vi "PI_AreaScan_Prepare_1.vi"(0 "System":i32 min=0 max=3 step=1, 1 "Laser":string, 2 "Axis":string, 3 "da":dbl min=-100.0 max=100.0, 4 "db":dbl min=-100.0 max=100.0, 5 "error in (no error)":errorcluster caption="Fehler (Eingang, kein Fehler)", 6 "a0":dbl min=2.0 max=198.0 step=0.01, 8 "b0":dbl min=0.0 max=200.0 step=0.01, 9 "Resolution":dbl min=0.01 max=2.0 step=0.01, 10 "c0":dbl min=0.0 max=200.0 step=0.01, 11 "Pixel time":dbl) -> (14 "Tacq":dbl, 15 "lp":i32, 16 "ap":i32, 17 "Trigger":dbl[](array[numeric]), 19 "error out":errorcluster caption="Fehler (Ausgang)")   [LabVIEW 2009]
panel:
  out "ClockDivider":i32
  out "Amplitude":dbl format="%#_3g"
  out "Accelaration":dbl
  out "ttp":i32
  out "Scan lines":dbl
  out "slow axis":i32
  out "fast axis":i32
  out "Colors":i32
  out "Start position":dbl[](array[numeric])
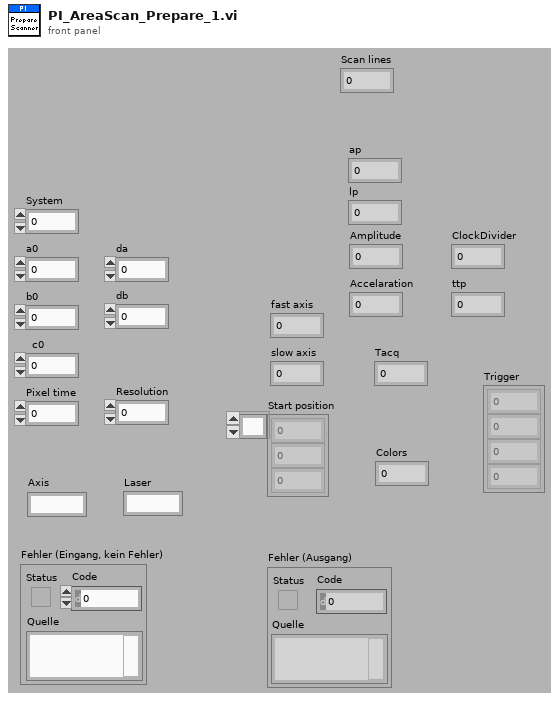
[diagram p1: front panel]
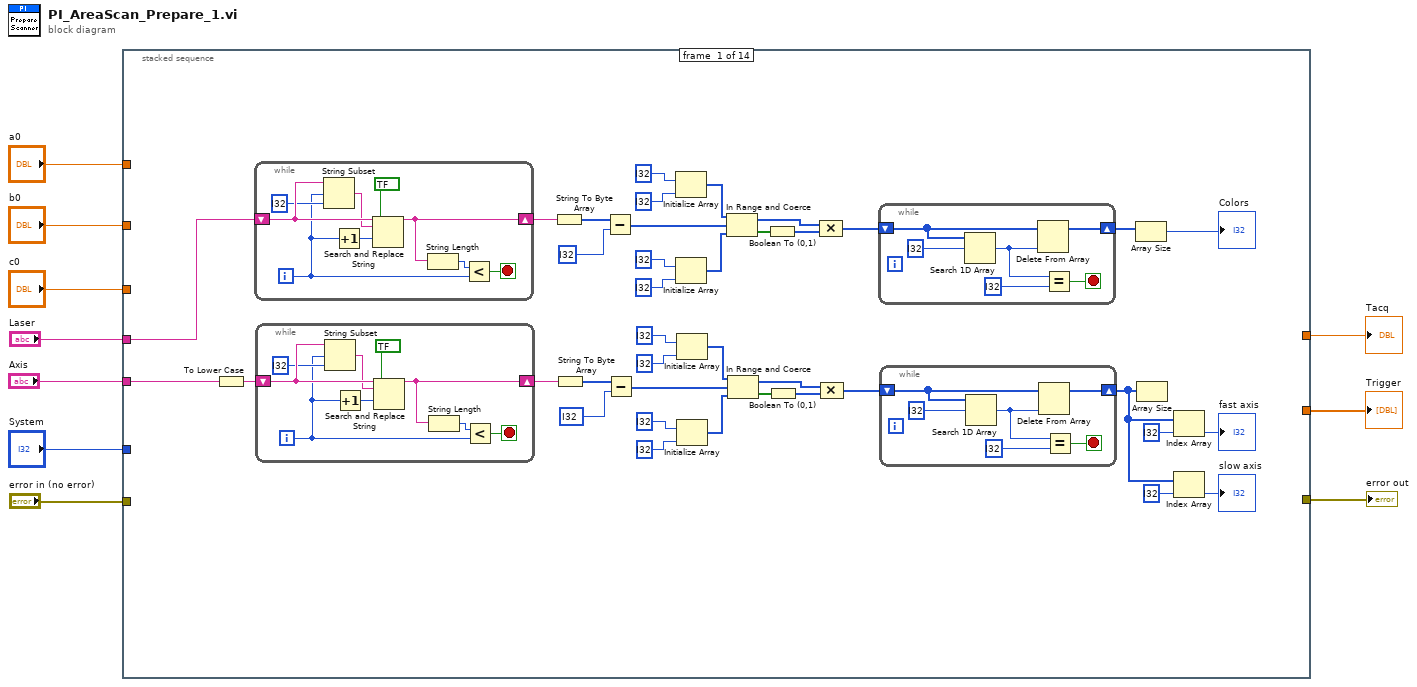
[diagram p0: block diagram]
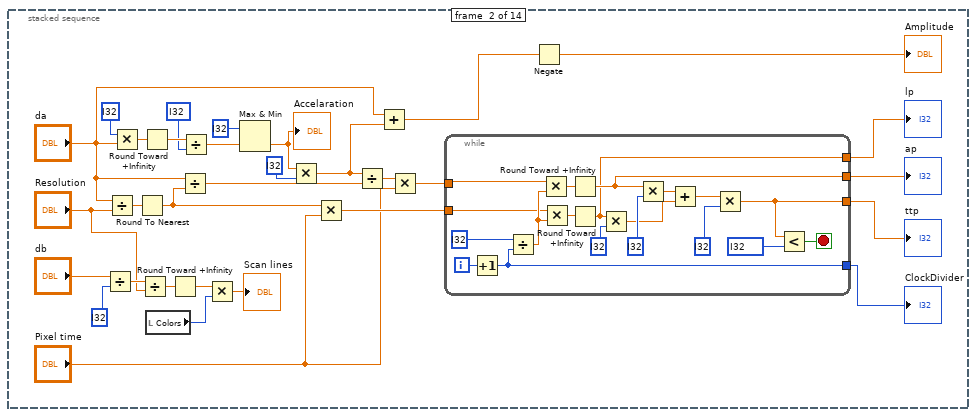
[diagram p2: hidden frame]
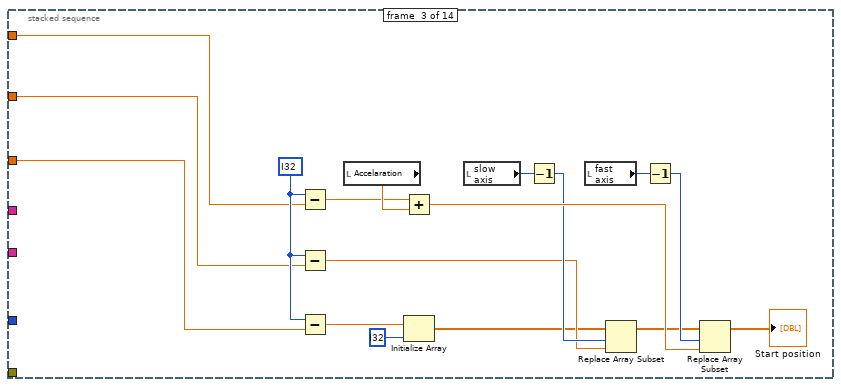
[diagram p3: hidden frame]
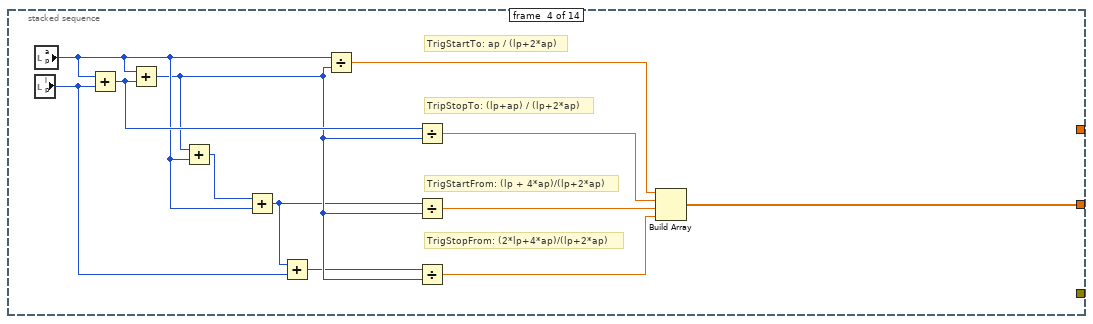
[diagram p4: hidden frame]
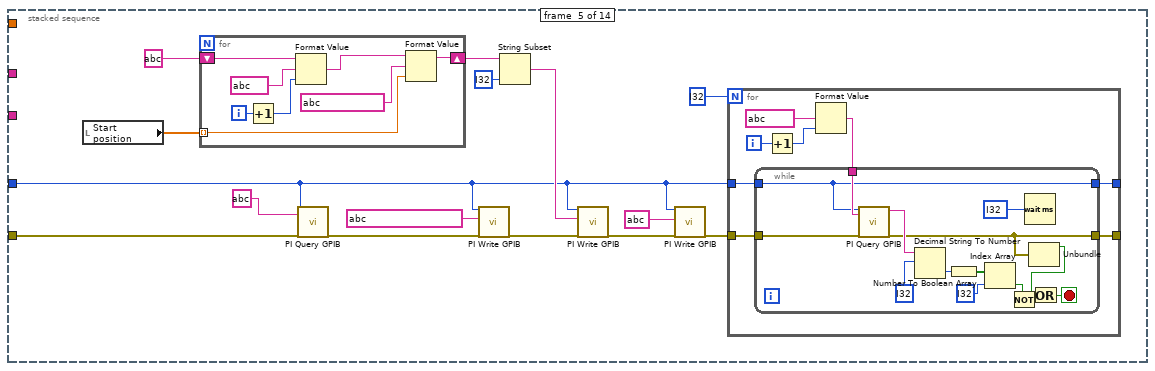
[diagram p5: hidden frame]
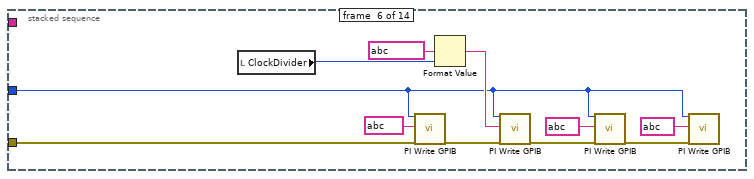
[diagram p6: hidden frame]
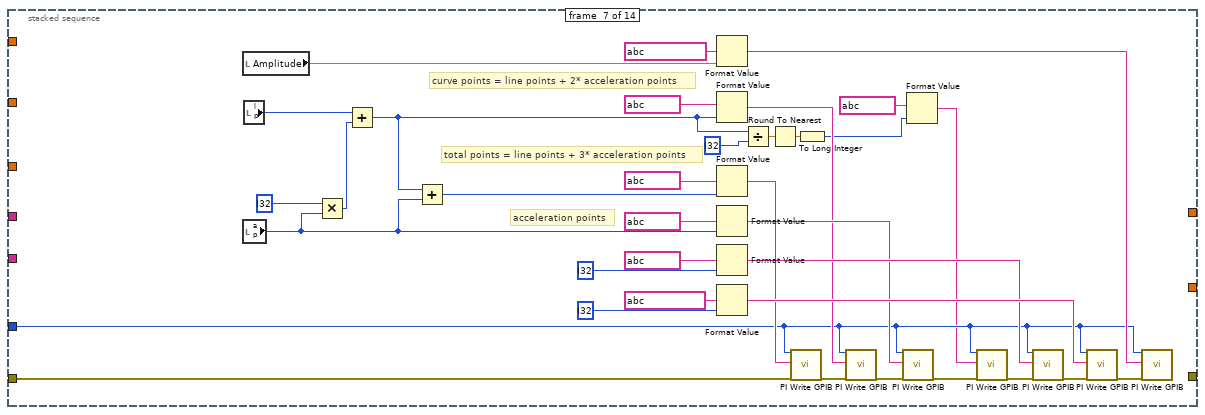
[diagram p7: hidden frame]
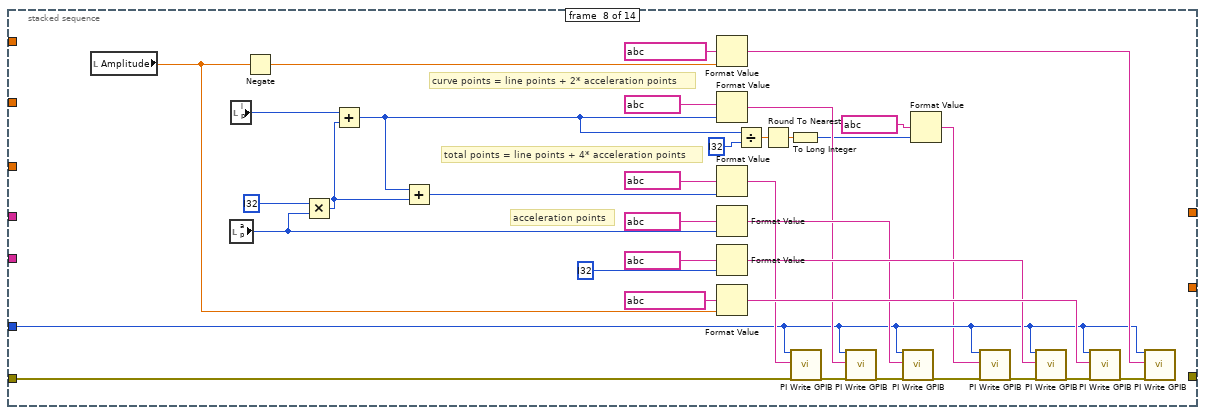
[diagram p8: hidden frame]
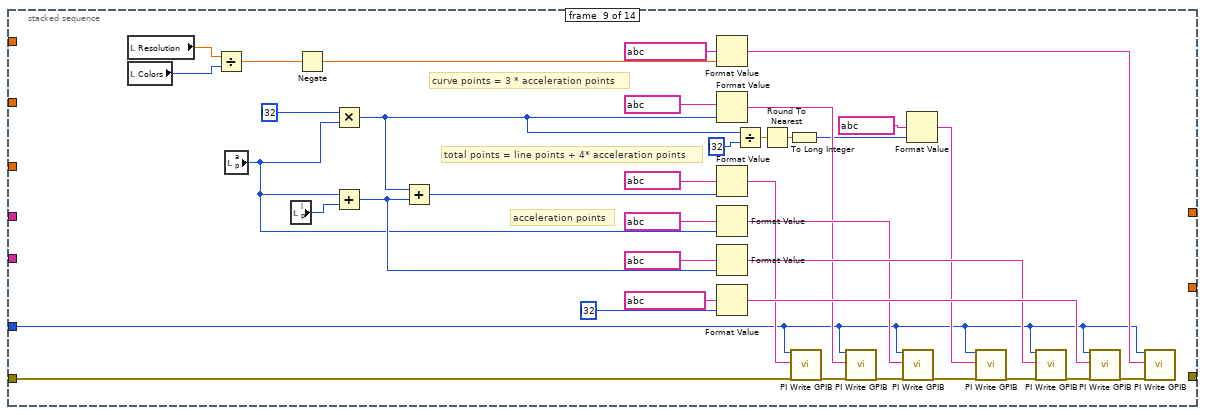
[diagram p9: hidden frame]
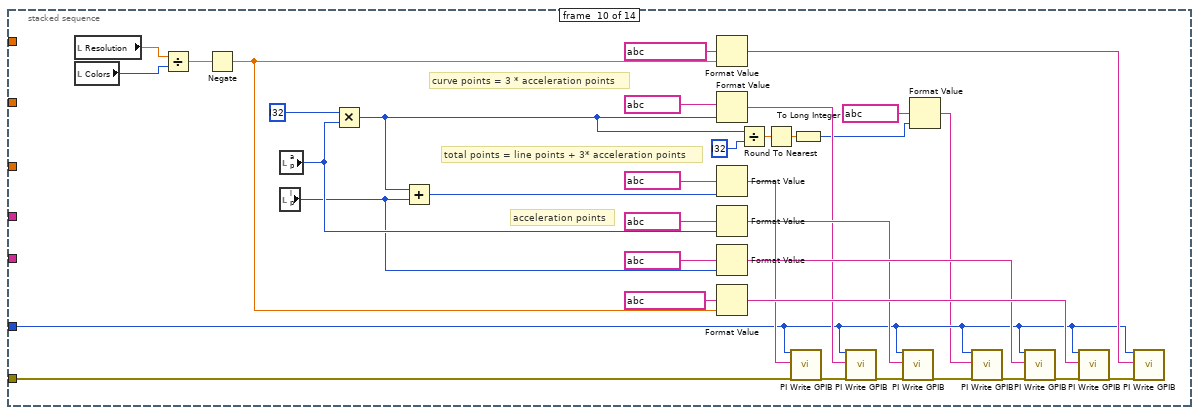
[diagram p10: hidden frame]
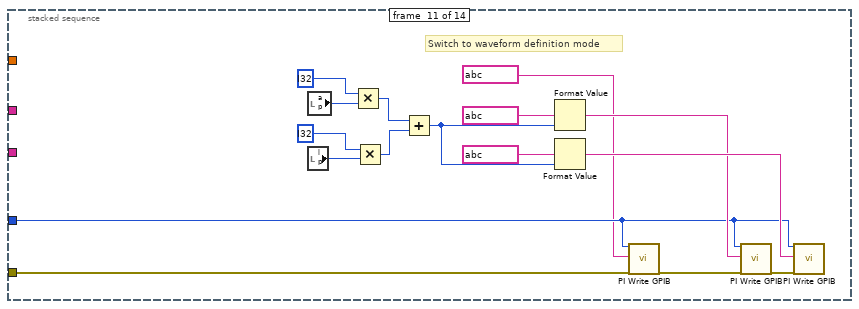
[diagram p11: hidden frame]
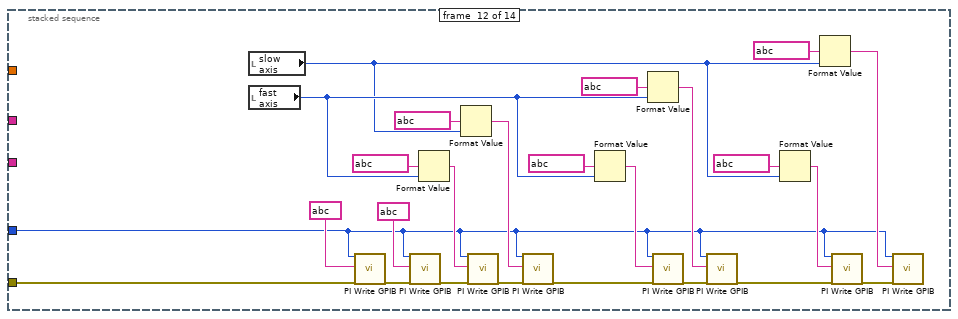
[diagram p12: hidden frame]
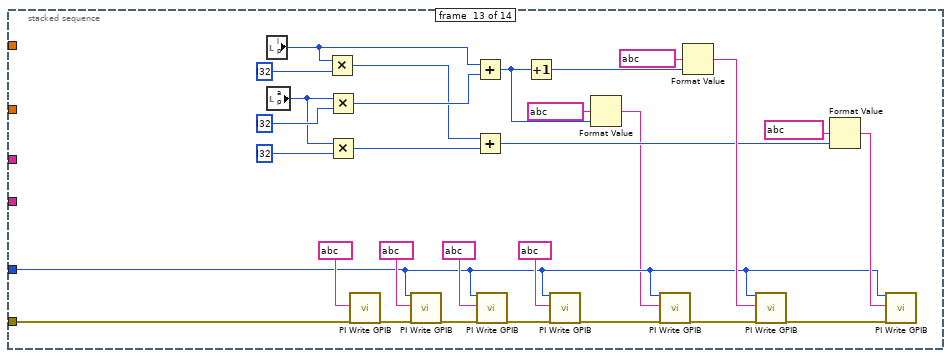
[diagram p13: hidden frame]
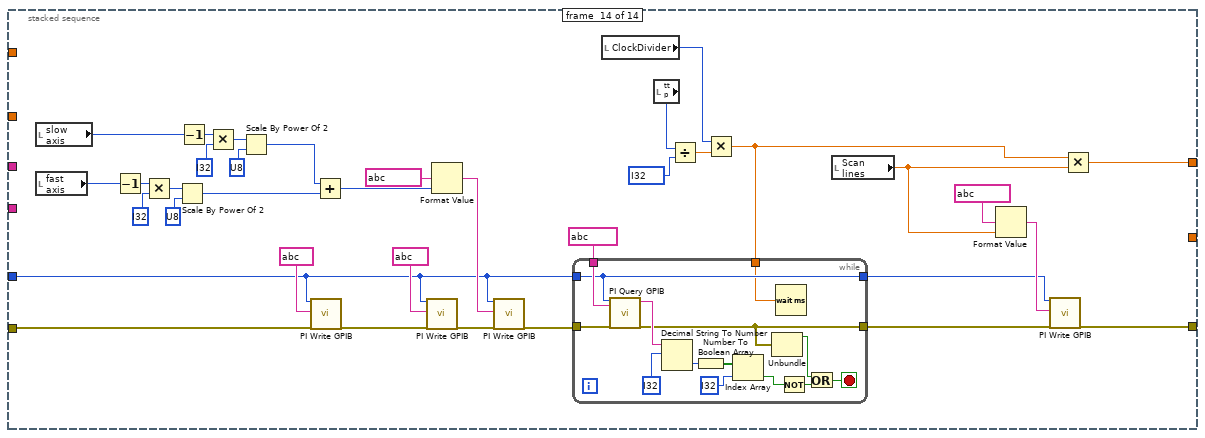
[diagram p14: hidden frame]
diagram:
  n1 = stacked-sequence {
    tunnel: "System" -> [_ _ _ _ w161 w203 w216 w254 w284 w324 w365 w372 w400 w427]
    tunnel: "error in (no error)" -> [_ _ _ _ w163 w204 w229 w266 w304 w339 w366 w373 w413 w428]
    tunnel: [_ _ _ _ _ _ _ _ _ _ _ _ _ w429] -> w8
    tunnel: "Laser" -> [w12 _ _ _ _ _ _ _ _ _ _ _ _ _]
    tunnel: "Axis" -> [w11 _ _ _ _ _ _ _ _ _ _ _ _ _]
    tunnel: "c0" -> [_ _ w131 _ _ _ _ _ _ _ _ _ _ _]
    tunnel: "b0" -> [_ _ w130 _ _ _ _ _ _ _ _ _ _ _]
    tunnel: "a0" -> [_ _ w129 _ _ _ _ _ _ _ _ _ _ _]
    tunnel: [_ _ _ _ _ _ _ _ _ _ _ _ _ w426] -> w2
    tunnel: [_ _ _ w146 _ _ _ _ _ _ _ _ _ _] -> w1
    frame #0 {
      n2 = To Lower Case(string=w11) -> (all lower case string=w19:string)
      n3 = while {
        shift-right: [w74] -> w39
        shift-left: w12 -> [w78]
        i -> [w70]
        stop <- w73 stop-if-true
        n4 = String Subset(string=w78, offset (0)=w70, length (rest)=i32 ?) -> (substring=w76:string)
        n5 = Increment(x=w70) -> (x+1=w71:i32)
        n6 = Search and Replace String(replace all?=bool ?, input string=w78, search string=w76, offset=w71) -> (result string=w74:string)  [unwired: 4 in, 3 out]
        n7 = String Length(string=w74) -> (length=w72:i32)
        n8 = Less?(x=w72, y=w70) -> (x < y?=w73:bool)
      }
      n9 = while {
        shift-right: [w59] -> w24
        shift-left: w19 -> [w63]
        i -> [w55]
        stop <- w58 stop-if-true
        n10 = String Subset(string=w63, offset (0)=w55, length (rest)=i32 ?) -> (substring=w61:string)
        n11 = Increment(x=w55) -> (x+1=w56:i32)
        n12 = Search and Replace String(replace all?=bool ?, input string=w63, search string=w61, offset=w56) -> (result string=w59:string)  [unwired: 4 in, 3 out]
        n13 = String Length(string=w59) -> (length=w57:i32)
        n14 = Less?(x=w57, y=w55) -> (x < y?=w58:bool)
      }
      n15 = String To Byte Array(string=w39) -> (unsigned byte array=w41:u8[])
      n16 = String To Byte Array(string=w24) -> (unsigned byte array=w26:u8[])
      n17 = Subtract(x=w41, y=i32 ?) -> (x-y=w38:i32[])
      n18 = Subtract(x=w26, y=i32 ?) -> (x-y=w23:i32[])
      n19 = Initialize Array(i32 ?, i32 ?) -> (w46:i32[])
      n20 = Initialize Array(i32 ?, i32 ?) -> (w43:i32[])
      n21 = Initialize Array(i32 ?, i32 ?) -> (w31:i32[])
      n22 = Initialize Array(i32 ?, i32 ?) -> (w28:i32[])
      n23 = In Range and Coerce(upper limit=w46, x=w38, lower limit=w43) -> (coerced(x)=w35:i32[], In Range?=w42:bool[])
      n24 = In Range and Coerce(upper limit=w31, x=w23, lower limit=w28) -> (coerced(x)=w20:i32[], In Range?=w27:bool[])
      n25 = Boolean To (0,1)(Boolean=w42) -> (0, 1=w36:i16[])
      n26 = Boolean To (0,1)(Boolean=w27) -> (0, 1=w21:i16[])
      n27 = Compound Arithmetic op=MULTIPLY(w35, w36) -> (w37:i32[])
      n28 = Compound Arithmetic op=MULTIPLY(w20, w21) -> (w22:i32[])
      n29 = while {
        shift-right: [w66] -> w34
        shift-left: w37 -> [w64]
        stop <- w67 stop-if-true
        n30 = Search 1D Array(1D array=w64, element=i32 ?) -> (index of element=w68:i32)  [unwired: 1 in]
        n31 = Delete From Array(array=w64, index=w68) -> (array with subset deleted=w66:i32[])  [unwired: 1 in, 1 out]
        n32 = Equal?(x=w68, y=i32 ?) -> (x = y?=w67:bool)
      }
      n33 = while {
        shift-right: [w51] -> w16
        shift-left: w22 -> [w49]
        stop <- w52 stop-if-true
        n34 = Search 1D Array(1D array=w49, element=i32 ?) -> (index of element=w53:i32)  [unwired: 1 in]
        n35 = Delete From Array(array=w49, index=w53) -> (array with subset deleted=w51:i32[])  [unwired: 1 in, 1 out]
        n36 = Equal?(x=w53, y=i32 ?) -> (x = y?=w52:bool)
      }
      n37 = Array Size(array=w34) -> (size(s)=→"Colors":i32)
      n38 = Array Size(array=w16) -> ()  [unwired: 1 out]
      n39 = Index Array(array=w16, index=i32 ?) -> (element=→"fast axis":i32)
      n40 = Index Array(array=w16, index=i32 ?) -> (element=→"slow axis":i32)
    }
    frame #1 {
      n41 = Divide(x="db", y=i32 ?) -> (x/y=w101:dbl)
      n42 = Divide(x="da", y="Resolution") -> (x/y=w103:dbl)
      n43 = Multiply(x=i32 ?, y="da") -> (x*y=w108:dbl)
      n44 = Round To Nearest(number=w103) -> (nearest integer value=w90:dbl)
      n45 = Divide(x=w101, y="Resolution") -> (x/y=w95:dbl)
      n46 = Round Toward +Infinity(x=w108) -> (ceil(x): smallest int >= x=w107:dbl)
      n47 = local read "Colors"() -> (w98:i32)
      n48 = Round Toward +Infinity(x=w95) -> (ceil(x): smallest int >= x=w96:dbl)
      n49 = Divide(x="da", y=w90) -> (x/y=w89:dbl)
      n50 = Divide(x=w107, y=i32 ?) -> (x/y=w105:dbl)
      n51 = Multiply(x=w96, y=w98) -> (x*y=→"Scan lines":dbl)
      n52 = Max & Min(x=i32 ?, y=w105) -> (min(x,y)=w86:dbl)  [unwired: 1 out]
      "Accelaration" <- w86
      n53 = Multiply(x=w86, y=i32 ?) -> (x*y=w88:dbl)
      n54 = Multiply(x=w90, y="Pixel time") -> (x*y=w94:dbl)
      n55 = Divide(x=w88, y=w89) -> (x/y=w91:dbl)
      n56 = Add(x="da", y=w88) -> (x+y=w80:dbl)
      n57 = Multiply(x=w91, y="Pixel time") -> (x*y=w92:dbl)
      n58 = while {
        tunnel: w94 -> [w125]
        tunnel: w92 -> [w124]
        tunnel: [w113] -> w84
        tunnel: [w112] -> w81
        tunnel: [w111] -> w83
        tunnel: [w110] -> w82
        i -> [w128]
        stop <- w114 stop-if-true
        n59 = Increment(x=w128) -> (x+1=w112:i32)
        n60 = Divide(x=i32 ?, y=w112) -> (x/y=w126:dbl)
        n61 = Multiply(x=w124, y=w126) -> (x*y=w123:dbl)
        n62 = Multiply(x=w125, y=w126) -> (x*y=w122:dbl)
        n63 = Round Toward +Infinity(x=w123) -> (ceil(x): smallest int >= x=w111:dbl)
        n64 = Round Toward +Infinity(x=w122) -> (ceil(x): smallest int >= x=w110:dbl)
        n65 = Multiply(x=w110, y=i32 ?) -> (x*y=w118:dbl)
        n66 = Multiply(x=w111, y=i32 ?) -> (x*y=w119:dbl)
        n67 = Add(x=w119, y=w118) -> (x+y=w117:dbl)
        n68 = Multiply(x=w117, y=i32 ?) -> (x*y=w113:dbl)
        n69 = Less?(x=w113, y=i32 ?) -> (x < y?=w114:bool)
      }
      "ttp" <- w84
      "ap" <- w83
      "lp" <- w82
      "ClockDivider" <- w81
      n70 = Negate(x=w80) -> (-x=→"Amplitude":dbl)
    }
    frame #2 {
      w132 = i32 ?
      n71 = Subtract(x=w132, y=w129) -> (x-y=w140:dbl)
      n72 = Subtract(x=w132, y=w130) -> (x-y=w136:dbl)
      n73 = Subtract(x=w132, y=w131) -> (x-y=w134:dbl)
      n74 = local read "Accelaration"() -> (w142:dbl)
      n75 = Add(x=w140, y=w142) -> (x+y=w141:dbl)
      n76 = Initialize Array(w134, i32 ?) -> (w135:dbl[])
      n77 = local read "slow axis"() -> (w145:i32)
      n78 = Decrement(x=w145) -> (x-1=w138:i32)
      n79 = local read "fast axis"() -> (w144:i32)
      n80 = Replace Array Subset(array=w135, new element=w136, index=w138) -> (w137:dbl[])
      n81 = Decrement(x=w144) -> (x-1=w139:i32)
      n82 = Replace Array Subset(array=w137, new element=w141, index=w139) -> (→"Start position":dbl[])
    }
    frame #3 {
      # "TrigStopFrom: (2*lp+4*ap)/(lp+2*ap)"
      # "TrigStartFrom: (lp + 4*ap)/(lp+2*ap)"
      # "TripStopTo: (lp+ap) / (lp+2*ap)"
      # "TrigStartTo: ap / (lp+2*ap)"
      n83 = local read "ap"() -> (w152:i32)
      n84 = local read "lp"() -> (w148:i32)
      n85 = Add(x=w152, y=w148) -> (x+y=w153:i32)
      n86 = Add(x=w152, y=w153) -> (x+y=w151:i32)
      n87 = Add(x=w151, y=w152) -> (x+y=w150:i32)
      n88 = Add(x=w150, y=w152) -> (x+y=w147:i32)
      n89 = Add(x=w147, y=w148) -> (x+y=w149:i32)
      n90 = Divide(x=w152, y=w151) -> (x/y=w154:dbl)
      n91 = Divide(x=w153, y=w151) -> (x/y=w155:dbl)
      n92 = Divide(x=w147, y=w151) -> (x/y=w156:dbl)
      n93 = Divide(x=w149, y=w151) -> (x/y=w157:dbl)
      n94 = Build Array(w154, w155, w156, w157) -> (w146:dbl[])
    }
    frame #4 {
      n95 = local read "Start position"() -> (w160:dbl[])
      n96 = for {
        shift-right: [w200] -> w170
        shift-left: string ? -> [w202]
        tunnel: w160 -> [w195] mode=indexing
        i -> [w197]
        n97 = Increment(x=w197) -> (x+1=w196:i32)
        n98 = Format Value(string ("")=w202, format string=string ?, value (0)=w196) -> (output string=w201:string)
        n99 = Format Value(string ("")=w201, format string=string ?, value (0)=w195) -> (output string=w200:string)
      }
      n100 = call "PI Query GPIB.vi"("System no."=w161, "String to send"=string ?, "error in"=w163) -> ("error out"=w168:errorcluster)  [unwired: 14 in, 2 out]
      n101 = call "PI Write GPIB.vi"("System no."=w161, "String to send"=string ?, "error in"=w168) -> ("error out"=w164:errorcluster)  [unwired: 16 in]
      n102 = String Subset(string=w170, length (rest)=i32 ?) -> (substring=w172:string)  [unwired: 1 in]
      n103 = call "PI Write GPIB.vi"("System no."=w161, "String to send"=w172, "error in"=w164) -> ("error out"=w166:errorcluster)  [unwired: 16 in]
      n104 = call "PI Write GPIB.vi"("System no."=w161, "String to send"=string ?, "error in"=w166) -> ("error out"=w165:errorcluster)  [unwired: 16 in]
      n105 = for {
        N: i32 ? -> [_]
        tunnel: w165 -> [w176]
        tunnel: w161 -> [w175]
        tunnel: [w174] -> _
        tunnel: [w173] -> _
        i -> [w180]
        n106 = Increment(x=w180) -> (x+1=w179:i32)
        n107 = Format Value(format string=string ?, value (0)=w179) -> (output string=w177:string)  [unwired: 1 in]
        n108 = while {
          tunnel: w177 -> [w194]
          tunnel: w176 -> [w193]
          tunnel: w175 -> [w189]
          tunnel: [w188] -> w174
          tunnel: [w189] -> w173
          stop <- w183 stop-if-true
          n109 = call "PI Query GPIB.vi"("System no."=w189, "String to send"=w194, "error in"=w193) -> ("String read"=w191:string, "error out"=w188:errorcluster)  [unwired: 14 in, 1 out]
          n110 = Decimal String To Number(string=w191, offset=i32 ?) -> (number=w190:i32)  [unwired: 1 in, 1 out]
          n111 = Number To Boolean Array(number=w190) -> (Boolean array=w185:bool[])
          n112 = Index Array(array=w185, index=i32 ?) -> (element=w184:bool)
          n113 = Not(x=w184) -> (.not. x?=w181:bool)
          n114 = Wait (ms)(milliseconds to wait=i32 ?) -> ()  [unwired: 1 out]
          n115 = Unbundle(w188) -> ("status"=w187:bool)  [unwired: 2 out]
          n116 = Or(x=w187, y=w181) -> (x .or. y?=w183:bool)
        }
      }
    }
    frame #5 {
      n117 = local read "ClockDivider"() -> (w213:i32)
      n118 = call "PI Write GPIB.vi"("System no."=w203, "String to send"=string ?, "error in"=w204) -> ("error out"=w205:errorcluster)  [unwired: 16 in]
      n119 = Format Value(format string=string ?, value (0)=w213) -> (output string=w210:string)  [unwired: 1 in]
      n120 = call "PI Write GPIB.vi"("System no."=w203, "String to send"=w210, "error in"=w205) -> ("error out"=w207:errorcluster)  [unwired: 16 in]
      n121 = call "PI Write GPIB.vi"("System no."=w203, "String to send"=string ?, "error in"=w207) -> ("error out"=w208:errorcluster)  [unwired: 16 in]
      n122 = call "PI Write GPIB.vi"("System no."=w203, "String to send"=string ?, "error in"=w208) -> ()  [unwired: 16 in, 1 out]
    }
    frame #6 {
      # "acceleration points"
      # "total points = line points + 3* acceleration points"
      # "curve points = line points + 2* acceleration points"
      n123 = local read "Amplitude"() -> (w214:dbl)
      n124 = local read "ap"() -> (w225:i32)
      n125 = local read "lp"() -> (w227:i32)
      n126 = Multiply(x=i32 ?, y=w225) -> (x*y=w228:i32)
      n127 = Add(x=w227, y=w228) -> (x+y=w222:i32)
      n128 = Add(x=w222, y=w225) -> (x+y=w226:i32)
      n129 = Format Value(format string=string ?, value (0)=w214) -> (output string=w247:string)  [unwired: 1 in]
      n130 = Format Value(format string=string ?, value (0)=w222) -> (output string=w243:string)  [unwired: 1 in]
      n131 = Format Value(format string=string ?, value (0)=w226) -> (output string=w242:string)  [unwired: 1 in]
      n132 = Format Value(format string=string ?, value (0)=w225) -> (output string=w244:string)  [unwired: 1 in]
      n133 = Format Value(format string=string ?, value (0)=i32 ?) -> (output string=w245:string)  [unwired: 1 in]
      n134 = Format Value(format string=string ?, value (0)=i32 ?) -> (output string=w246:string)  [unwired: 1 in]
      n135 = Divide(x=w222, y=i32 ?) -> (x/y=w221:dbl)
      n136 = Round To Nearest(number=w221) -> (nearest integer value=w218:dbl)
      n137 = call "PI Write GPIB.vi"("System no."=w216, "String to send"=w242, "error in"=w229) -> ("error out"=w241:errorcluster)  [unwired: 16 in]
      n138 = To Long Integer(number=w218) -> (32bit integer=w219:i32)
      n139 = call "PI Write GPIB.vi"("System no."=w216, "String to send"=w243, "error in"=w241) -> ("error out"=w248:errorcluster)  [unwired: 16 in]
      n140 = call "PI Write GPIB.vi"("System no."=w216, "String to send"=w244, "error in"=w248) -> ("error out"=w238:errorcluster)  [unwired: 16 in]
      n141 = Format Value(format string=string ?, value (0)=w219) -> (output string=w215:string)  [unwired: 1 in]
      n142 = call "PI Write GPIB.vi"("System no."=w216, "String to send"=w215, "error in"=w238) -> ("error out"=w217:errorcluster)  [unwired: 16 in]
      n143 = call "PI Write GPIB.vi"("System no."=w216, "String to send"=w245, "error in"=w217) -> ("error out"=w239:errorcluster)  [unwired: 16 in]
      n144 = call "PI Write GPIB.vi"("System no."=w216, "String to send"=w246, "error in"=w239) -> ("error out"=w240:errorcluster)  [unwired: 16 in]
      n145 = call "PI Write GPIB.vi"("System no."=w216, "String to send"=w247, "error in"=w240) -> ()  [unwired: 16 in, 1 out]
    }
    frame #7 {
      # "acceleration points"
      # "total points = line points + 4* acceleration points"
      # "curve points = line points + 2* acceleration points"
      n146 = local read "Amplitude"() -> (w250:dbl)
      n147 = local read "ap"() -> (w263:i32)
      n148 = local read "lp"() -> (w265:i32)
      n149 = Negate(x=w250) -> (-x=w249:dbl)
      n150 = Multiply(x=i32 ?, y=w263) -> (x*y=w262:i32)
      n151 = Add(x=w265, y=w262) -> (x+y=w252:i32)
      n152 = Add(x=w252, y=w262) -> (x+y=w264:i32)
      n153 = Format Value(format string=string ?, value (0)=w249) -> (output string=w282:string)  [unwired: 1 in]
      n154 = Format Value(format string=string ?, value (0)=w252) -> (output string=w278:string)  [unwired: 1 in]
      n155 = Format Value(format string=string ?, value (0)=w264) -> (output string=w277:string)  [unwired: 1 in]
      n156 = Format Value(format string=string ?, value (0)=w263) -> (output string=w279:string)  [unwired: 1 in]
      n157 = Format Value(format string=string ?, value (0)=i32 ?) -> (output string=w280:string)  [unwired: 1 in]
      n158 = Format Value(format string=string ?, value (0)=w250) -> (output string=w281:string)  [unwired: 1 in]
      n159 = Divide(x=w252, y=i32 ?) -> (x/y=w260:dbl)
      n160 = Round To Nearest(number=w260) -> (nearest integer value=w257:dbl)
      n161 = To Long Integer(number=w257) -> (32bit integer=w258:i32)
      n162 = call "PI Write GPIB.vi"("System no."=w254, "String to send"=w277, "error in"=w266) -> ("error out"=w276:errorcluster)  [unwired: 16 in]
      n163 = call "PI Write GPIB.vi"("System no."=w254, "String to send"=w278, "error in"=w276) -> ("error out"=w283:errorcluster)  [unwired: 16 in]
      n164 = call "PI Write GPIB.vi"("System no."=w254, "String to send"=w279, "error in"=w283) -> ("error out"=w256:errorcluster)  [unwired: 16 in]
      n165 = Format Value(format string=string ?, value (0)=w258) -> (output string=w253:string)  [unwired: 1 in]
      n166 = call "PI Write GPIB.vi"("System no."=w254, "String to send"=w253, "error in"=w256) -> ("error out"=w255:errorcluster)  [unwired: 16 in]
      n167 = call "PI Write GPIB.vi"("System no."=w254, "String to send"=w280, "error in"=w255) -> ("error out"=w274:errorcluster)  [unwired: 16 in]
      n168 = call "PI Write GPIB.vi"("System no."=w254, "String to send"=w281, "error in"=w274) -> ("error out"=w275:errorcluster)  [unwired: 16 in]
      n169 = call "PI Write GPIB.vi"("System no."=w254, "String to send"=w282, "error in"=w275) -> ()  [unwired: 16 in, 1 out]
    }
    frame #8 {
      # "acceleration points"
      # "total points = line points + 4* acceleration points"
      # "curve points = 3 * acceleration points"
      n170 = local read "Resolution"() -> (w302:dbl)
      n171 = local read "Colors"() -> (w299:i32)
      n172 = Divide(x=w302, y=w299) -> (x/y=w300:dbl)
      n173 = local read "ap"() -> (w294:i32)
      n174 = local read "lp"() -> (w297:i32)
      n175 = Negate(x=w300) -> (-x=w298:dbl)
      n176 = Multiply(x=i32 ?, y=w294) -> (x*y=w289:i32)
      n177 = Add(x=w294, y=w297) -> (x+y=w295:i32)
      n178 = Add(x=w289, y=w295) -> (x+y=w303:i32)
      n179 = Format Value(format string=string ?, value (0)=w298) -> (output string=w319:string)  [unwired: 1 in]
      n180 = Format Value(format string=string ?, value (0)=w289) -> (output string=w315:string)  [unwired: 1 in]
      n181 = Format Value(format string=string ?, value (0)=w303) -> (output string=w314:string)  [unwired: 1 in]
      n182 = Format Value(format string=string ?, value (0)=w294) -> (output string=w316:string)  [unwired: 1 in]
      n183 = Format Value(format string=string ?, value (0)=w295) -> (output string=w317:string)  [unwired: 1 in]
      n184 = Format Value(format string=string ?, value (0)=i32 ?) -> (output string=w318:string)  [unwired: 1 in]
      n185 = Divide(x=w289, y=i32 ?) -> (x/y=w293:dbl)
      n186 = Round To Nearest(number=w293) -> (nearest integer value=w290:dbl)
      n187 = To Long Integer(number=w290) -> (32bit integer=w291:i32)
      n188 = call "PI Write GPIB.vi"("System no."=w284, "String to send"=w314, "error in"=w304) -> ("error out"=w313:errorcluster)  [unwired: 16 in]
      n189 = call "PI Write GPIB.vi"("System no."=w284, "String to send"=w315, "error in"=w313) -> ("error out"=w320:errorcluster)  [unwired: 16 in]
      n190 = call "PI Write GPIB.vi"("System no."=w284, "String to send"=w316, "error in"=w320) -> ("error out"=w286:errorcluster)  [unwired: 16 in]
      n191 = Format Value(format string=string ?, value (0)=w291) -> (output string=w287:string)  [unwired: 1 in]
      n192 = call "PI Write GPIB.vi"("System no."=w284, "String to send"=w287, "error in"=w286) -> ("error out"=w285:errorcluster)  [unwired: 16 in]
      n193 = call "PI Write GPIB.vi"("System no."=w284, "String to send"=w317, "error in"=w285) -> ("error out"=w311:errorcluster)  [unwired: 16 in]
      n194 = call "PI Write GPIB.vi"("System no."=w284, "String to send"=w318, "error in"=w311) -> ("error out"=w312:errorcluster)  [unwired: 16 in]
      n195 = call "PI Write GPIB.vi"("System no."=w284, "String to send"=w319, "error in"=w312) -> ()  [unwired: 16 in, 1 out]
    }
    frame #9 {
      # "acceleration points"
      # "total points = line points + 3* acceleration points"
      # "curve points = 3 * acceleration points"
      n196 = local read "Resolution"() -> (w337:dbl)
      n197 = local read "Colors"() -> (w336:i32)
      n198 = Divide(x=w337, y=w336) -> (x/y=w333:dbl)
      n199 = Negate(x=w333) -> (-x=w331:dbl)
      n200 = local read "ap"() -> (w334:i32)
      n201 = local read "lp"() -> (w332:i32)
      n202 = Multiply(x=i32 ?, y=w334) -> (x*y=w322:i32)
      n203 = Add(x=w322, y=w332) -> (x+y=w338:i32)
      n204 = Format Value(format string=string ?, value (0)=w331) -> (output string=w354:string)  [unwired: 1 in]
      n205 = Format Value(format string=string ?, value (0)=w322) -> (output string=w350:string)  [unwired: 1 in]
      n206 = Format Value(format string=string ?, value (0)=w338) -> (output string=w349:string)  [unwired: 1 in]
      n207 = Format Value(format string=string ?, value (0)=w334) -> (output string=w351:string)  [unwired: 1 in]
      n208 = Format Value(format string=string ?, value (0)=w332) -> (output string=w352:string)  [unwired: 1 in]
      n209 = Format Value(format string=string ?, value (0)=w331) -> (output string=w353:string)  [unwired: 1 in]
      n210 = Divide(x=w322, y=i32 ?) -> (x/y=w330:dbl)
      n211 = Round To Nearest(number=w330) -> (nearest integer value=w327:dbl)
      n212 = call "PI Write GPIB.vi"("System no."=w324, "String to send"=w349, "error in"=w339) -> ("error out"=w348:errorcluster)  [unwired: 16 in]
      n213 = To Long Integer(number=w327) -> (32bit integer=w328:i32)
      n214 = call "PI Write GPIB.vi"("System no."=w324, "String to send"=w350, "error in"=w348) -> ("error out"=w355:errorcluster)  [unwired: 16 in]
      n215 = call "PI Write GPIB.vi"("System no."=w324, "String to send"=w351, "error in"=w355) -> ("error out"=w326:errorcluster)  [unwired: 16 in]
      n216 = Format Value(format string=string ?, value (0)=w328) -> (output string=w323:string)  [unwired: 1 in]
      n217 = call "PI Write GPIB.vi"("System no."=w324, "String to send"=w323, "error in"=w326) -> ("error out"=w325:errorcluster)  [unwired: 16 in]
      n218 = call "PI Write GPIB.vi"("System no."=w324, "String to send"=w352, "error in"=w325) -> ("error out"=w346:errorcluster)  [unwired: 16 in]
      n219 = call "PI Write GPIB.vi"("System no."=w324, "String to send"=w353, "error in"=w346) -> ("error out"=w347:errorcluster)  [unwired: 16 in]
      n220 = call "PI Write GPIB.vi"("System no."=w324, "String to send"=w354, "error in"=w347) -> ()  [unwired: 16 in, 1 out]
    }
    frame #10 {
      # "Switch to waveform definition mode"
      n221 = local read "ap"() -> (w361:i32)
      n222 = local read "lp"() -> (w362:i32)
      n223 = Multiply(x=i32 ?, y=w361) -> (x*y=w358:i32)
      n224 = Multiply(x=i32 ?, y=w362) -> (x*y=w357:i32)
      n225 = Add(x=w358, y=w357) -> (x+y=w356:i32)
      n226 = Format Value(format string=string ?, value (0)=w356) -> (output string=w370:string)  [unwired: 1 in]
      n227 = Format Value(format string=string ?, value (0)=w356) -> (output string=w371:string)  [unwired: 1 in]
      n228 = call "PI Write GPIB.vi"("System no."=w365, "String to send"=string ?, "error in"=w366) -> ("error out"=w363:errorcluster)  [unwired: 16 in]
      n229 = call "PI Write GPIB.vi"("System no."=w365, "String to send"=w370, "error in"=w363) -> ("error out"=w369:errorcluster)  [unwired: 16 in]
      n230 = call "PI Write GPIB.vi"("System no."=w365, "String to send"=w371, "error in"=w369) -> ()  [unwired: 16 in, 1 out]
    }
    frame #11 {
      n231 = local read "slow axis"() -> (w387:i32)
      n232 = local read "fast axis"() -> (w388:i32)
      n233 = call "PI Write GPIB.vi"("System no."=w372, "String to send"=string ?, "error in"=w373) -> ("error out"=w379:errorcluster)  [unwired: 16 in]
      n234 = call "PI Write GPIB.vi"("System no."=w372, "String to send"=string ?, "error in"=w379) -> ("error out"=w374:errorcluster)  [unwired: 16 in]
      n235 = Format Value(format string=string ?, value (0)=w388) -> (output string=w391:string)  [unwired: 1 in]
      n236 = Format Value(format string=string ?, value (0)=w387) -> (output string=w392:string)  [unwired: 1 in]
      n237 = call "PI Write GPIB.vi"("System no."=w372, "String to send"=w391, "error in"=w374) -> ("error out"=w375:errorcluster)  [unwired: 16 in]
      n238 = call "PI Write GPIB.vi"("System no."=w372, "String to send"=w392, "error in"=w375) -> ("error out"=w376:errorcluster)  [unwired: 16 in]
      n239 = Format Value(format string=string ?, value (0)=w388) -> (output string=w393:string)  [unwired: 1 in]
      n240 = Format Value(format string=string ?, value (0)=w388) -> (output string=w394:string)  [unwired: 1 in]
      n241 = call "PI Write GPIB.vi"("System no."=w372, "String to send"=w393, "error in"=w376) -> ("error out"=w377:errorcluster)  [unwired: 16 in]
      n242 = call "PI Write GPIB.vi"("System no."=w372, "String to send"=w394, "error in"=w377) -> ("error out"=w378:errorcluster)  [unwired: 16 in]
      n243 = Format Value(format string=string ?, value (0)=w387) -> (output string=w395:string)  [unwired: 1 in]
      n244 = Format Value(format string=string ?, value (0)=w387) -> (output string=w396:string)  [unwired: 1 in]
      n245 = call "PI Write GPIB.vi"("System no."=w372, "String to send"=w395, "error in"=w378) -> ("error out"=w386:errorcluster)  [unwired: 16 in]
      n246 = call "PI Write GPIB.vi"("System no."=w372, "String to send"=w396, "error in"=w386) -> ()  [unwired: 16 in, 1 out]
    }
    frame #12 {
      n247 = local read "lp"() -> (w407:i32)
      n248 = local read "ap"() -> (w409:i32)
      n249 = Multiply(x=w407, y=i32 ?) -> (x*y=w405:i32)
      n250 = Multiply(x=w409, y=i32 ?) -> (x*y=w412:i32)
      n251 = Multiply(x=w409, y=i32 ?) -> (x*y=w406:i32)
      n252 = call "PI Write GPIB.vi"("String to send"=string ?, "error in"=w413) -> ("error out"=w415:errorcluster)  [unwired: 17 in]
      n253 = call "PI Write GPIB.vi"("System no."=w400, "String to send"=string ?, "error in"=w415) -> ("error out"=w414:errorcluster)  [unwired: 16 in]
      n254 = Add(x=w407, y=w412) -> (x+y=w397:i32)
      n255 = Add(x=w405, y=w406) -> (x+y=w404:i32)
      n256 = call "PI Write GPIB.vi"("System no."=w400, "String to send"=string ?, "error in"=w414) -> ("error out"=w417:errorcluster)  [unwired: 16 in]
      n257 = Increment(x=w397) -> (x+1=w398:i32)
      n258 = call "PI Write GPIB.vi"("System no."=w400, "String to send"=string ?, "error in"=w417) -> ("error out"=w416:errorcluster)  [unwired: 16 in]
      n259 = Format Value(format string=string ?, value (0)=w397) -> (output string=w399:string)  [unwired: 1 in]
      n260 = call "PI Write GPIB.vi"("System no."=w400, "String to send"=w399, "error in"=w416) -> ("error out"=w401:errorcluster)  [unwired: 16 in]
      n261 = Format Value(format string=string ?, value (0)=w398) -> (output string=w423:string)  [unwired: 1 in]
      n262 = call "PI Write GPIB.vi"("System no."=w400, "String to send"=w423, "error in"=w401) -> ("error out"=w403:errorcluster)  [unwired: 16 in]
      n263 = Format Value(format string=string ?, value (0)=w404) -> (output string=w425:string)  [unwired: 1 in]
      n264 = call "PI Write GPIB.vi"("System no."=w400, "String to send"=w425, "error in"=w403) -> ()  [unwired: 16 in, 1 out]
    }
    frame #13 {
      n265 = local read "slow axis"() -> (w459:i32)
      n266 = local read "fast axis"() -> (w458:i32)
      n267 = Decrement(x=w458) -> (x-1=w439:i32)
      n268 = Multiply(x=w439, y=i32 ?) -> (x*y=w437:i32)
      n269 = Scale By Power Of 2(n=w437, x=u8 ?) -> (x*2^n=w441:u8)
      n270 = Decrement(x=w459) -> (x-1=w435:i32)
      n271 = Multiply(x=w435, y=i32 ?) -> (x*y=w433:i32)
      n272 = Scale By Power Of 2(n=w433, x=u8 ?) -> (x*2^n=w440:u8)
      n273 = call "PI Write GPIB.vi"("System no."=w427, "String to send"=string ?, "error in"=w428) -> ("error out"=w460:errorcluster)  [unwired: 16 in]
      n274 = Add(x=w440, y=w441) -> (x+y=w442:u8)
      n275 = call "PI Write GPIB.vi"("System no."=w427, "String to send"=string ?, "error in"=w460) -> ("error out"=w430:errorcluster)  [unwired: 16 in]
      n276 = Format Value(format string=string ?, value (0)=w442) -> (output string=w454:string)  [unwired: 1 in]
      n277 = call "PI Write GPIB.vi"("System no."=w427, "String to send"=w454, "error in"=w430) -> ("error out"=w443:errorcluster)  [unwired: 16 in]
      n278 = local read "ClockDivider"() -> (w457:i32)
      n279 = local read "ttp"() -> (w456:i32)
      n280 = Divide(x=w456, y=i32 ?) -> (x/y=w445:dbl)
      n281 = Multiply(x=w457, y=w445) -> (x*y=w448:dbl)
      n282 = while {
        tunnel: string ? -> [w474]
        tunnel: w443 -> [w473]
        tunnel: w427 -> [w469]
        tunnel: [w464] -> w451
        tunnel: [w469] -> w450
        tunnel: w448 -> [w468]
        stop <- w465 stop-if-true
        n283 = call "PI Query GPIB.vi"("System no."=w469, "String to send"=w474, "error in"=w473) -> ("String read"=w471:string, "error out"=w464:errorcluster)  [unwired: 14 in, 1 out]
        n284 = Decimal String To Number(string=w471, offset=i32 ?) -> (number=w470:i32)  [unwired: 1 in, 1 out]
        n285 = Number To Boolean Array(number=w470) -> (Boolean array=w467:bool[])
        n286 = Index Array(array=w467, index=i32 ?) -> (element=w463:bool)
        n287 = Unbundle(w464) -> ("status"=w462:bool)  [unwired: 2 out]
        n288 = Wait (ms)(milliseconds to wait=w468) -> ()  [unwired: 1 out]
        n289 = Not(x=w463) -> (.not. x?=w461:bool)
        n290 = Or(x=w462, y=w461) -> (x .or. y?=w465:bool)
      }
      n291 = local read "Scan lines"() -> (w447:dbl)
      n292 = Format Value(format string=string ?, value (0)=w447) -> (output string=w455:string)  [unwired: 1 in]
      n293 = call "PI Write GPIB.vi"("System no."=w450, "String to send"=w455, "error in"=w451) -> ("error out"=w429:errorcluster)  [unwired: 16 in]
      n294 = Multiply(x=w448, y=w447) -> (x*y=w426:dbl)
    }
  }
  "error out" <- w8
  "Tacq" <- w2
  "Trigger" <- w1
